vi "Read.vi"(8 "error in (no error)":errorcluster, 11 "Two Terminal in":refnum<class "AbsFunc_Two Term_STR.lvclass">) -> (0 "error out":errorcluster, 2 "String":string, 3 "Two Terminal out":refnum<class "AbsFunc_Two Term_STR.lvclass">)   [LabVIEW 2021, in "AbsFunc_Two Term_STR.lvclass"]
uses:
  AbsFunc_Two Term_STR.lvclass
  AbsFunc_Two Term_STR.lvclass/AbsFunc_Two Term_STR.ctl
  Abs_Types/String/Abs_String.lvclass
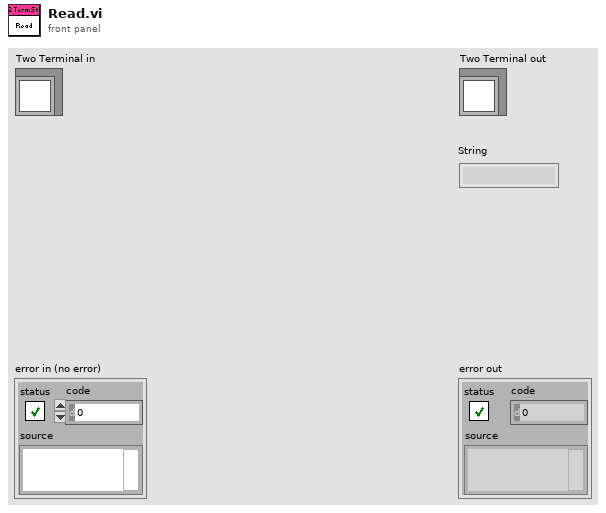
[diagram p1: front panel]
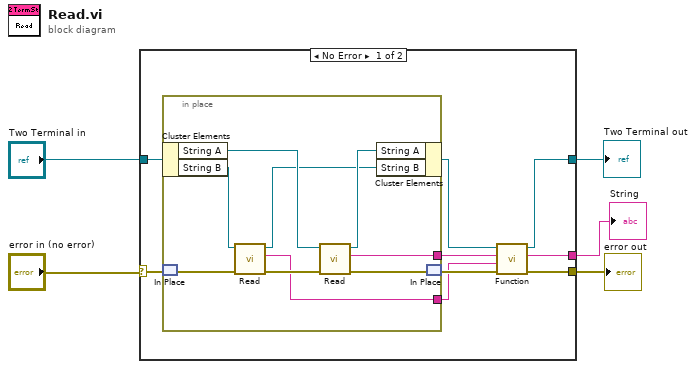
[diagram p0: block diagram]
diagram:
  n1 = case shown="No Error" "error in (no error)" {
    selector: "error in (no error)" -> [w13 w24]
    tunnel: "Two Terminal in" -> [w14 w25]
    tunnel: [w7 w24] -> w3
    tunnel: [w8 w25] -> w2
    tunnel: [w6 _] -> w1
    frame No Error {
      n2 = in-place {
        in-place-border: [w20] -> w10
        in-place-border: [w15] -> w9
        n3 = in-place-cluster #1(w14) -> ("String A"=w22:refnum<class "Abs_String.lvclass">, "String B"=w17:refnum<class "Abs_String.lvclass">)
        n4 = in-place-match #2(w13) -> (w19:errorcluster)
        n5 = call-dynamic "Read.vi"("error in (no error)"=w19, "Abs_String in"=w17) -> ("error out"=w18:errorcluster, "String"=w15:string, "Abs_String out"=w16:refnum<class "Abs_String.lvclass">)  [unwired: 7 in]
        n6 = call-dynamic "Read.vi"("error in (no error)"=w18, "Abs_String in"=w22) -> ("error out"=w23:errorcluster, "String"=w20:string, "Abs_String out"=w21:refnum<class "Abs_String.lvclass">)  [unwired: 7 in]
        n7 = in-place-cluster #1("String A"=w21, "String B"=w16) -> (w12:refnum<class "AbsFunc_Two Term_STR.lvclass">)
        n8 = in-place-match #2(w23) -> (w11:errorcluster)
      }
      n9 = call-dynamic "Function.vi"("error in (no error)"=w11, "String B"=w9, "String A"=w10, "Two Terminal in"=w12) -> ("error out"=w7:errorcluster, "Result"=w6:string, "Two Terminal out"=w8:refnum<class "AbsFunc_Two Term_STR.lvclass">)  [unwired: 5 in]
    }
    frame Error {
    }
  }
  "error out" <- w3
  "Two Terminal out" <- w2
  "String" <- w1
